vi "Custom waveform signal generation.vi"() -> ()   [LabVIEW 2010]
doc: "This example shows how to program Red Pitaya to generate custom waveform signal. Red Pitaya is able to generate signals in range from DC to 50 MHz with output voltage range from -1 to 1 Volt. Generated signal can be observed by Red Pitaya Oscilloscope WEB application. To run it, just open web browser, input Red Pitaya IP and start Oscilloscope."
uses:
  RedPitaya.lvlib
panel:
  out "Waveform Graph 2":dbl[](graph)
  out "Waveform Graph 1":dbl[](graph)
  in  "IP address":string="192.168.1.100"
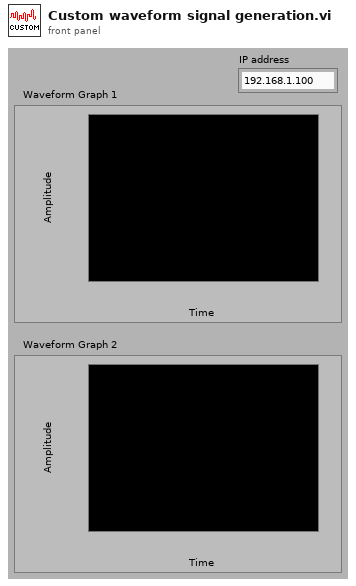
[diagram p1: front panel]
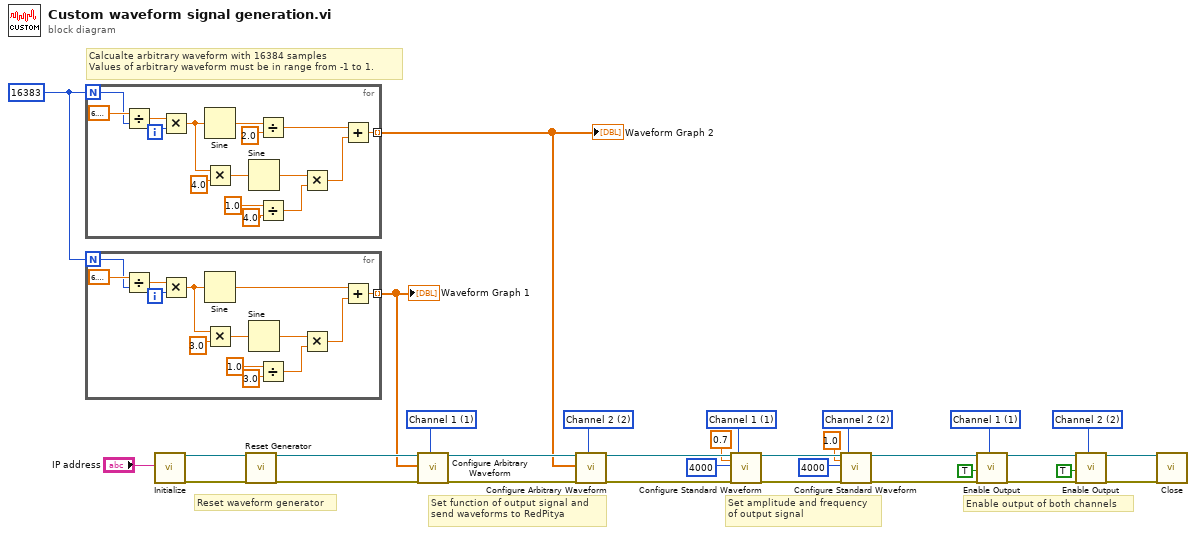
[diagram p0: block diagram]
diagram:
  w7 = u16 2 items=["Channel 1"=1, "Channel 2"=2] ("Channel #")
  w17 = u16 2 items=["Channel 1"=1, "Channel 2"=2] ("Channel (1|2)")
  w18 = u16 1 items=["Channel 1"=1, "Channel 2"=2] ("Channel (1|2)")
  w5 = 2 items=["Channel 1"=1, "Channel 2"=2] ("Channel (0: 1)")
  w30 = 16383
  w6 = 1 items=["Channel 1"=1, "Channel 2"=2] ("Channel (0: 1)")
  w4 = u16 1 items=["Channel 1"=1, "Channel 2"=2] ("Channel (1|2)")
  # "Reset waveform generator"
  # "Enable output of both channels"
  # "Set amplitude and frequency\nof output signal"
  # "Set function of output signal and\nsend waveforms to RedPitya"
  # "Calcualte arbitrary waveform with 16384 samples\nValues of arbitrary waveform must be in range from -1 to 1."
  n1 = for {
    N: w30 -> [w39]
    tunnel: [w40] -> w9 mode=indexing
    i -> [w37]
    n2 = Divide(x=6.283185307179586, y=w39) -> (x/y=w38:dbl)
    n3 = Multiply(x=w38, y=w37) -> (x*y=w36:dbl)
    n4 = Sine(x=w36) -> (sin(x)=w35:dbl)
    n5 = Multiply(x=w36, y=4.0) -> (x*y=w46:dbl)
    n6 = Sine(x=w46) -> (sin(x)=w43:dbl)
    n7 = Divide(x=w35, y=2.0) -> (x/y=w33:dbl)
    n8 = Divide(x=1.0, y=4.0) -> (x/y=w42:dbl)
    n9 = Multiply(x=w43, y=w42) -> (x*y=w41:dbl)
    n10 = Add(x=w33, y=w41) -> (x+y=w40:dbl)
  }
  "Waveform Graph 2" <- w9
  n11 = for {
    N: w30 -> [w52]
    tunnel: [w53] -> w8 mode=indexing
    i -> [w50]
    n12 = Divide(x=6.283185307179586, y=w52) -> (x/y=w51:dbl)
    n13 = Multiply(x=w51, y=w50) -> (x*y=w49:dbl)
    n14 = Sine(x=w49) -> (sin(x)=w55:dbl)
    n15 = Multiply(x=w49, y=3.0) -> (x*y=w60:dbl)
    n16 = Sine(x=w60) -> (sin(x)=w57:dbl)
    n17 = Divide(x=1.0, y=3.0) -> (x/y=w56:dbl)
    n18 = Multiply(x=w57, y=w56) -> (x*y=w54:dbl)
    n19 = Add(x=w55, y=w54) -> (x+y=w53:dbl)
  }
  "Waveform Graph 1" <- w8
  n20 = call "Initialize.vi"("IP address"="IP address") -> ("RedPitaya TCP Connection"=w12:refnum<k5>, "error out"=w10:errorcluster)  [unwired: 17 in]
  n21 = call "Reset Generator.vi"("RedPitaya connection in"=w12, "error in"=w10) -> ("RedPitaya connection out"=w11:refnum<k5>, "error out"=w3:errorcluster)  [unwired: 16 in]
  n22 = call "Configure Arbitrary Waveform.vi"("RedPitaya connection in"=w11, "Data"=w8, "error in"=w3, "Channel #"=w4) -> ("RedPitaya connection out"=w29:refnum<k5>, "error out"=w2:errorcluster)  [unwired: 14 in]
  n23 = call "Configure Arbitrary Waveform.vi"("RedPitaya connection in"=w29, "Data"=w9, "error in"=w2, "Channel #"=w7) -> ("RedPitaya connection out"=w23:refnum<k5>, "error out"=w1:errorcluster)  [unwired: 14 in]
  n24 = call "Configure Standard Waveform.vi"("RedPitaya connection in"=w23, "Amplitude"=0.7, "Frequency"=4000 ("Frequency (1000 Hz)"), "error in"=w1, "Channel #"=w18) -> ("RedPitaya connection out"=w22:refnum<k5>, "error out"=w19:errorcluster)  [unwired: 13 in]
  n25 = call "Configure Standard Waveform.vi"("RedPitaya connection in"=w22, "Amplitude"=1.0, "Frequency"=4000 ("Frequency (1000 Hz)"), "error in"=w19, "Channel #"=w17) -> ("RedPitaya connection out"=w21:refnum<k5>, "error out"=w20:errorcluster)  [unwired: 13 in]
  n26 = call "Enable Output.vi"("RedPitaya connection in"=w21, "Generation (T: Enable)"=TRUE, "error in"=w20, "Channel #"=w6) -> ("RedPitaya connection out"=w28:refnum<k5>, "error out"=w27:errorcluster)  [unwired: 14 in]
  n27 = call "Enable Output.vi"("RedPitaya connection in"=w28, "Generation (T: Enable)"=TRUE, "error in"=w27, "Channel #"=w5) -> ("RedPitaya connection out"=w25:refnum<k5>, "error out"=w24:errorcluster)  [unwired: 14 in]
  n28 = call "Close.vi"("connection ID"=w25, "error in"=w24) -> ()  [unwired: 17 in, 1 out]
